vi "CloseLog.vi"(11 "logger":T1) -> ()   [LabVIEW 2019]
uses:
  Logger.ctl
  <vilib>/Utility/error.llb/DialogType.ctl
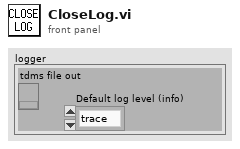
[diagram p1: front panel]
types:
  T1 = typedef "Logger.ctl" = cluster{"tdms file out":refnum<k34>, "Default log level (info)":enum16{"trace", "debug", "info", "warn", "error"}}
  T2 = typedef "DialogType.ctl" = u16
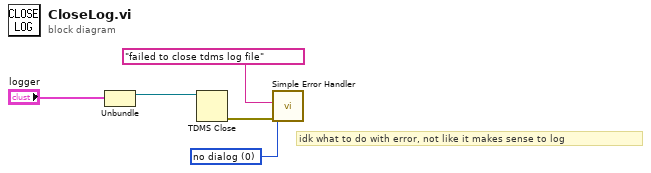
[diagram p0: block diagram]
diagram:
  w2 = T2 0 items=["no dialog", "OK message", "continue or stop message", "OK message + warnings", "continue/stop + warnings"] ("type of dialog (OK msg:1)")
  # "idk what to do with error, not like it makes sense to log"
  n1 = Unbundle("logger") -> ("tdms file out"=w5:refnum<k34>)  [unwired: 1 out]
  n2 = TDMS Close(11:w5) -> (0:w4:errorcluster)  [unwired: 1 in, 1 out]
  n3 = call <vilib>:"Simple Error Handler.vi"("error source (\" \")"="failed to close tdms log file" ("error source (\" \")"), "type of dialog (OK msg:1)"=w2, "error in (no error)"=w4) -> ()  [unwired: 2 in, 5 out]
